vi "valuePathv2.vi"(8 "error in (no error)":errorcluster, 9 "nodePath":string, 10 "value":string, 11 "xmlNode in":refnum<class "xmlNode.lvclass">) -> (0 "error out":errorcluster, 2 "Array":string[](array[string]), 3 "xmlNode out":refnum<class "xmlNode.lvclass">)   [LabVIEW 2011, in "Tools.lvlib" / "xml.lvlib" / "xmlNode.lvclass"]
doc: "please use valuePathv3 instead"
uses:
  xmlNode.lvclass
  XmlParser.lvclass
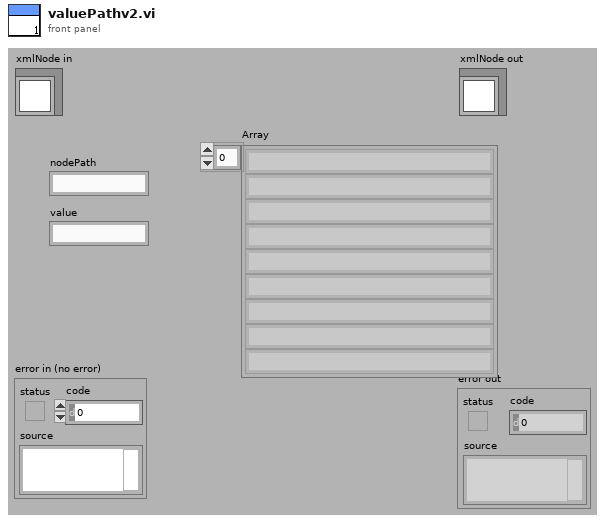
[diagram p1: front panel]
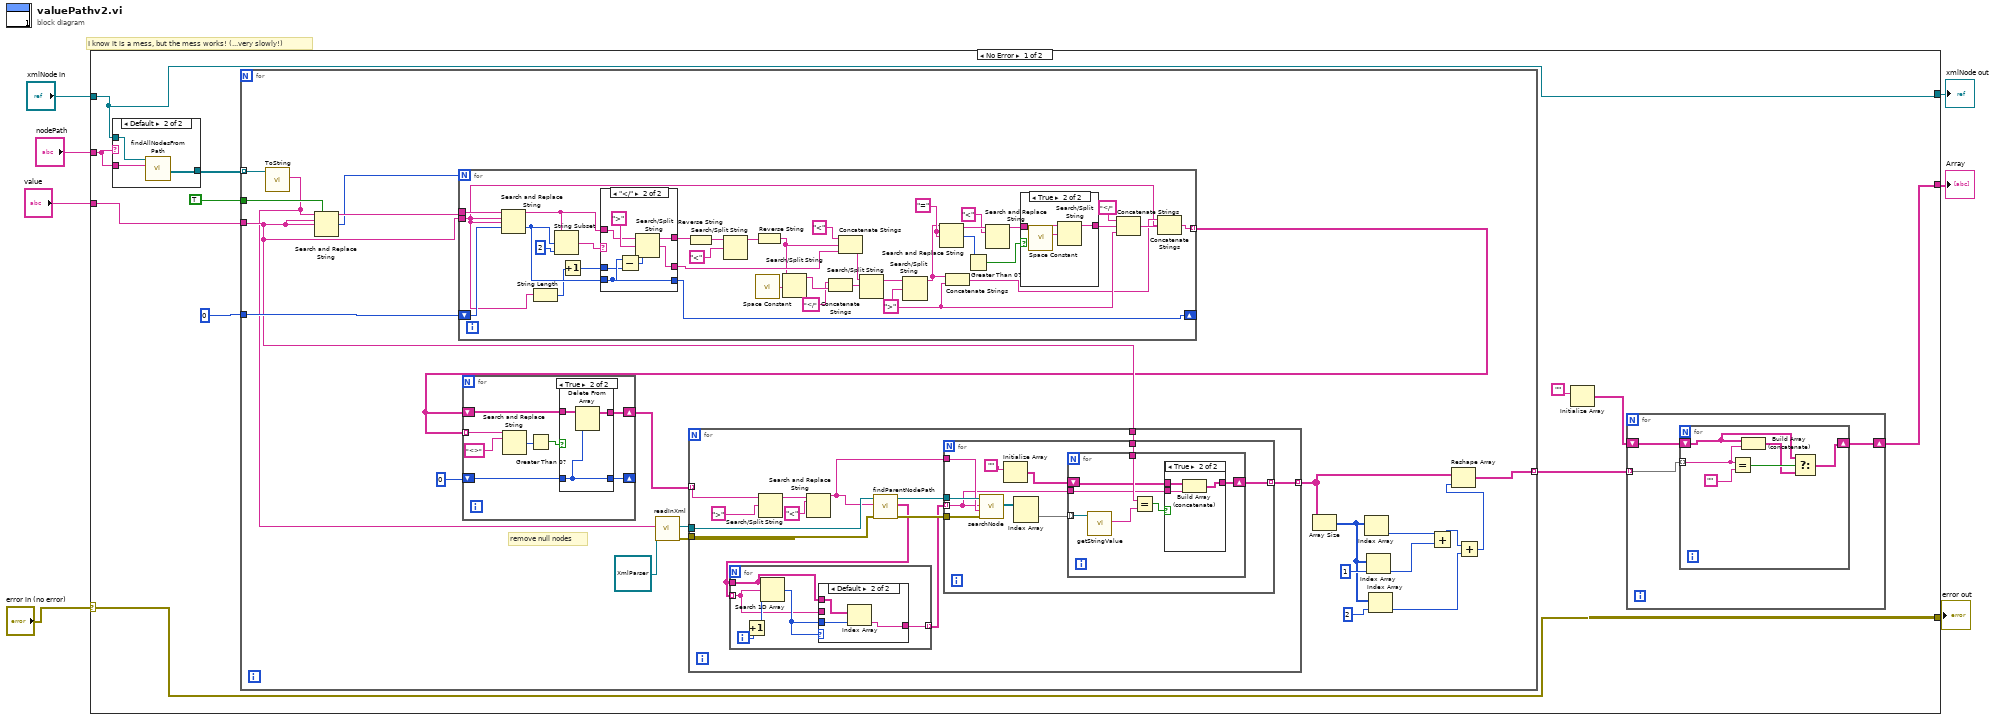
[diagram p0: block diagram]
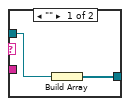
[diagram p2: hidden frame]
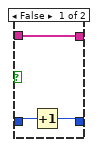
[diagram p5: hidden frame]
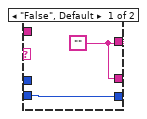
[diagram p7: hidden frame]
diagram:
  # "I know it is a mess, but the mess works! (...very slowly!)"
  n1 = case shown="No Error" "error in (no error)" {
    selector: "error in (no error)" -> [w9 w164]
    tunnel: [w9 w164] -> w6
    tunnel: [w11 w163] -> w4
    tunnel: "xmlNode in" -> [w11 w163]
    tunnel: "nodePath" -> [w8 _]
    tunnel: [w12 _] -> w2
    tunnel: "value" -> [w10 _]
    frame No Error {
      n2 = case shown="Default" w8 {
        tunnel: [w19 w23] -> w16
        tunnel: w8 -> [_ w22]
        tunnel: w11 -> [w20 w21]
        frame "" {
          n3 = Build Array(w20) -> (w19:refnum<class "xmlNode.lvclass">[])
        }
        frame Default {
          n4 = call "findAllNodesFromPath.vi"("nodePath"=w22, "xmlNode in"=w21) -> ("arrayXmlNodes"=w23:refnum<class "xmlNode.lvclass">[])  [unwired: 7 in, 2 out]
        }
      }
      n5 = for {
        tunnel: TRUE -> [w54]
        tunnel: 0 -> [w53]
        tunnel: w10 -> [w48]
        tunnel: w16 -> [w47] mode=indexing
        tunnel: [w45] -> w13 mode=indexing
        # "remove null nodes"
        n6 = call-dynamic "ToString.vi"("xmlNode in"=w47) -> ("xml"=w33:string)  [unwired: 8 in, 2 out]
        n7 = Search and Replace String(replace all?=w54, input string=w33, search string=w48, replace string=w48) -> (result string=w55:string, number of replacements=w44:i32)  [unwired: 4 in, 2 out]
        n8 = for {
          N: w44 -> [_]
          tunnel: w55 -> [w149]
          tunnel: w48 -> [w125]
          shift-right: [w115] -> _
          shift-left: w53 -> [w141]
          tunnel: [w133] -> w46 mode=indexing
          w139 = "="
          w135 = ">"
          n9 = Search and Replace String(input string=w149, search string=w125, replace string=w125, offset=w141) -> (result string=w145:string, offset past replacement=w146:i32)  [unwired: 4 in, 2 out]
          n10 = String Length(string=w125) -> (length=w124:i32)
          n11 = String Subset(string=w145, offset (0)=w146, length (rest)=2) -> (substring=w148:string)
          n12 = Increment(x=w124) -> (x+1=w123:i32)
          n13 = case shown="\"</\"" w148 {
            tunnel: w146 -> [w155 w158]
            tunnel: [w154 w160] -> w143
            tunnel: w145 -> [_ w161]
            tunnel: [w155 w158] -> w115
            tunnel: w123 -> [_ w157]
            tunnel: [w154 w156] -> w122
            frame "False", Default {
              w154 = ""
            }
            frame "</" {
              n14 = Subtract(x=w158, y=w157) -> (x-y=w159:i32)
              n15 = Search/Split String(string=w161, search string/char (-)=">", offset (0)=w159) -> (substring before match=w160:string, match + rest of string=w156:string)  [unwired: 1 out]
            }
          }
          n16 = Reverse String(1:w143) -> (0:w144:string)
          n17 = Search/Split String(string=w144, search string/char (-)="<") -> (substring before match=w142:string)  [unwired: 1 in, 2 out]
          n18 = call <vilib>:"Space Constant.vi"() -> ("String"=w119:string)
          n19 = Reverse String(1:w142) -> (0:w120:string)
          n20 = Search/Split String(string=w120, search string/char (-)=w119) -> (substring before match=w117:string)  [unwired: 1 in, 2 out]
          n21 = Concatenate Strings("</", w117) -> (w118:string)
          n22 = Concatenate Strings("<", w120, w122) -> (w121:string)
          n23 = Search/Split String(string=w121, search string/char (-)=w118) -> (substring before match=w114:string)  [unwired: 1 in, 2 out]
          n24 = Search/Split String(string=w114, search string/char (-)=w135) -> (substring before match=w131:string)  [unwired: 1 in, 2 out]
          n25 = Search and Replace String(input string=w131, search string=w139, replace string=w139) -> (result string=w127:string, number of replacements=w138:i32)  [unwired: 5 in, 2 out]
          n26 = Concatenate Strings(w131, w135) -> (w132:string)
          n27 = Greater Than 0?(x=w138) -> (x > 0?=w137:bool)
          n28 = Search and Replace String(input string=w127, search string="<") -> (result string=w128:string)  [unwired: 6 in, 3 out]
          n29 = case shown="True" w137 {
            tunnel: w128 -> [w150 w153]
            tunnel: [w150 w151] -> w136
            frame False {
            }
            frame True {
              n30 = call <vilib>:"Space Constant.vi"() -> ("String"=w152:string)
              n31 = Search/Split String(string=w153, search string/char (-)=w152) -> (substring before match=w151:string)  [unwired: 1 in, 2 out]
            }
          }
          n32 = Concatenate Strings("</", w136, w135) -> (w134:string)
          n33 = Concatenate Strings(w132, w125, w134) -> (w133:string)
        }
        n34 = for {
          tunnel: w46 -> [w107] mode=indexing
          shift-right: [w102] -> w51
          shift-left: w46 -> [w103]
          shift-right: [w100] -> _
          shift-left: 0 -> [w101]
          n35 = Search and Replace String(input string=w107, search string="<>") -> (number of replacements=w105:i32)  [unwired: 6 in, 3 out]
          n36 = Greater Than 0?(x=w105) -> (x > 0?=w104:bool)
          n37 = case shown="True" w104 {
            tunnel: w103 -> [w110 w113]
            tunnel: [w110 w112] -> w102
            tunnel: w101 -> [w109 w111]
            tunnel: [w108 w111] -> w100
            frame False {
              n38 = Increment(x=w109) -> (x+1=w108:i32)
            }
            frame True {
              n39 = Delete From Array(array=w113, index=w111) -> (array with subset deleted=w112:string[])  [unwired: 1 in, 1 out]
            }
          }
        }
        n40 = call "readInXml.vi"("xmlString"=w33, "XmlParser in"=refnum<class "XmlParser.lvclass"> refnum ("Tools.lvlib:xml.lvlib:XmlParser.lvclass")) -> ("error out"=w49:errorcluster, "xmlNode"=w34:refnum<class "xmlNode.lvclass">)  [unwired: 7 in, 1 out]
        n41 = for {
          tunnel: w51 -> [w66] mode=indexing
          tunnel: w34 -> [w68]
          tunnel: w49 -> [w67]
          tunnel: w48 -> [w59]
          tunnel: [w58] -> w43 mode=indexing
          n42 = Search/Split String(string=w66, search string/char (-)=">") -> (substring before match=w64:string)  [unwired: 1 in, 2 out]
          n43 = Search and Replace String(input string=w64, search string="<") -> (result string=w60:string)  [unwired: 6 in, 3 out]
          n44 = call-dynamic "findParentNodePath.vi"("error in (no error)"=w67, "searchElement"=w60, "xmlNode in"=w68) -> ("error out"=w61:errorcluster, "Paths"=w57:string[], "xmlNode out"=w62:refnum<class "xmlNode.lvclass">)  [unwired: 6 in]
          n45 = for {
            tunnel: w57 -> [w70] mode=indexing
            tunnel: [w74] -> w56 mode=indexing
            tunnel: w57 -> [w69]
            i -> [w73]
            n46 = Increment(x=w73) -> (x+1=w72:i32)
            n47 = Search 1D Array(1D array=w69, element=w70, start index (0)=w72) -> (index of element=w71:i32)
            n48 = case shown="Default" w71 {
              tunnel: w71 -> [_ w78]
              tunnel: [w75 w77] -> w74
              tunnel: w70 -> [w75 _]
              tunnel: w69 -> [_ w76]
              frame -1 {
              }
              frame Default {
                n49 = Index Array(array=w76, index=w78) -> (element=w77:string)
              }
            }
          }
          n50 = for {
            tunnel: w62 -> [w88]
            tunnel: w56 -> [w83] mode=indexing
            tunnel: w61 -> [w87]
            tunnel: w60 -> [w86]
            tunnel: w59 -> [w84]
            tunnel: [w80] -> w58 mode=indexing
            n51 = call-dynamic "searchNode.vi"("error in (no error)"=w87, "searchElementName"=w86, "searchElementIn"=w83, "xmlNode in"=w88) -> ("arrayXmlNodes"=w85:refnum<class "xmlNode.lvclass">[][])  [unwired: 5 in, 2 out]
            n52 = Initialize Array("") -> (w81:string[])  [unwired: 1 in]
            n53 = Index Array(array=w85) -> (element=w79:refnum<class "xmlNode.lvclass">[])  [unwired: 2 in]
            n54 = for {
              tunnel: w79 -> [w95] mode=indexing
              tunnel: w84 -> [w93]
              tunnel: w83 -> [w91]
              shift-right: [w90] -> w80
              shift-left: w81 -> [w89]
              n55 = call-dynamic "getStringValue.vi"("xmlNode.lvclass in"=w95) -> ("stringValue"=w94:string)  [unwired: 8 in, 2 out]
              n56 = Equal?(x=w93, y=w94) -> (x = y?=w92:bool)
              n57 = case shown="True" w92 {
                tunnel: w91 -> [_ w99]
                tunnel: [w96 w98] -> w90
                tunnel: w89 -> [w96 w97]
                frame False {
                }
                frame True {
                  n58 = Build Array (concatenate)(w97, w99) -> (w98:string[])
                }
              }
            }
          }
        }
        n59 = Array Size(array=w43) -> (size(s)=w39:i32[])
        n60 = Index Array(array=w39) -> (element=w40:i32)  [unwired: 1 in]
        n61 = Index Array(array=w39, index=1) -> (element=w41:i32)
        n62 = Index Array(array=w39, index=2) -> (element=w36:i32)
        n63 = Add(x=w40, y=w41) -> (x+y=w37:i32)
        n64 = Add(x=w37, y=w36) -> (x+y=w35:i32)
        n65 = Reshape Array(w43, w35) -> (w45:string[])
      }
      n66 = Initialize Array("") -> (w14:string[])  [unwired: 1 in]
      n67 = for {
        tunnel: w13 -> [w24] mode=indexing
        shift-right: [w26] -> w12
        shift-left: w14 -> [w25]
        n68 = for {
          tunnel: w24 -> [w30] mode=indexing
          shift-right: [w27] -> w26
          shift-left: w25 -> [w28]
          n69 = Equal?(x=w30, y="") -> (x = y?=w31:bool)
          n70 = Build Array (concatenate)(w28, w30) -> (w29:string[])
          n71 = Select(t=w28, s=w31, f=w29) -> (s? t:f=w27:string[])
        }
      }
    }
    frame Error {
    }
  }
  "error out" <- w6
  "xmlNode out" <- w4
  "Array" <- w2
